vi "srv_str2tcppack.vi"(8 "error in":errorcluster, 10 "string  in":string, 11 "connection ID":refnum<k5>) -> (0 "error out":errorcluster, 3 "connection ID out":refnum<k5>)   [LabVIEW 2013]
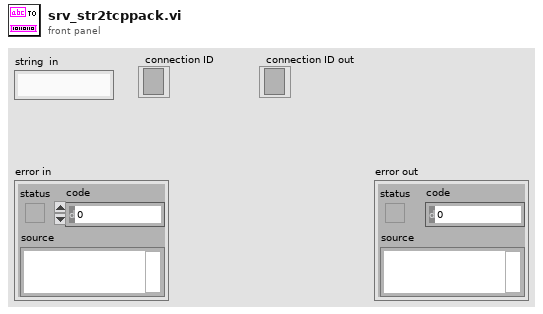
[diagram p1: front panel]
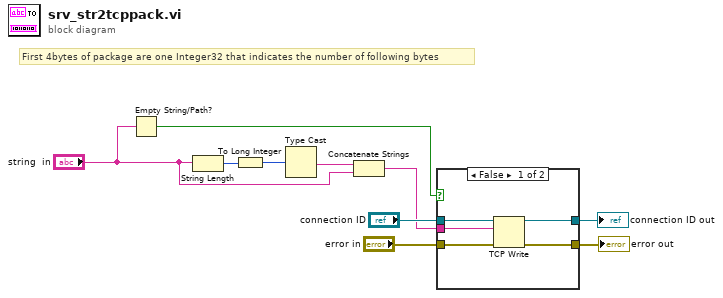
[diagram p0: block diagram]
diagram:
  # "First 4bytes of package are one Integer32 that indicates the number of following bytes"
  n1 = Empty String/Path?(string/path="string  in") -> (empty?=w1:bool)
  n2 = String Length(string="string  in") -> (length=w6:i32)
  n3 = To Long Integer(number=w6) -> (32bit integer=w5:i32)
  n4 = Type Cast(x=w5) -> (*(type *) &x=w4:string)  [unwired: 1 in]
  n5 = Concatenate Strings(w4, "string  in") -> (w3:string)
  n6 = case shown="False" w1 {
    tunnel: "connection ID" -> [w15 w17]
    tunnel: [w14 w17] -> w9
    tunnel: [w13 w16] -> w8
    tunnel: "error in" -> [w12 w16]
    tunnel: w3 -> [w11 _]
    frame False {
      n7 = TCP Write(connection ID=w15, data in=w11, error in (no error)=w12) -> (connection ID out=w14:refnum<k5>, error out=w13:errorcluster)  [unwired: 1 in, 1 out]
    }
    frame True {
    }
  }
  "error out" <- w8
  "connection ID out" <- w9
